vi "Measurement_WVFM.vi"(0 "dt":dbl, 2 "Input cluster":T1, 3 "Ioffset":dbl) -> (4 "Total power values":dbl[](array[numeric]), 5 "VL array":waveform(sgl)[](array[waveform]), 6 "VR array":waveform(sgl)[](array[waveform]), 7 "RMS values":dbl[](array[numeric]), 8 "Active Power":dbl[](array[numeric]))   [LabVIEW 2016]
uses:
  <vilib>/addons/Electrical Power/Basic/Measurement/RMS (N Channels).vi
  <vilib>/addons/Electrical Power/Basic/Measurement/Fundamental Vector (N Channels).vi
  <vilib>/addons/Electrical Power/Basic/NI_EP_Basic.lvlib
panel:
  out "RMS values I":dbl[](array[numeric])
  out "RMS values VR":dbl[](array[numeric])
  out "RMS values VL":dbl[](array[numeric])
  out "I array":waveform(sgl)[](array[waveform])
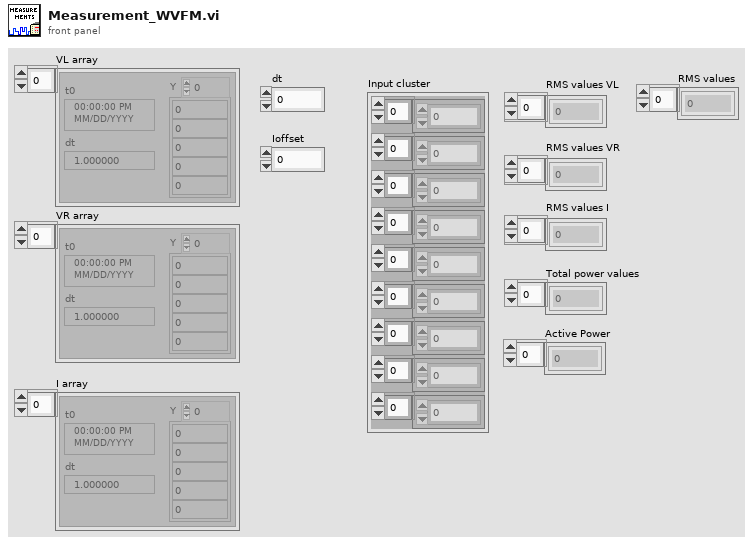
[diagram p1: front panel]
types:
  T1 = cluster{fxp<+/-,26,5>[], fxp<+/-,26,5>[], fxp<+/-,26,5>[], fxp<+/-,26,5>[], fxp<+/-,26,5>[], fxp<+/-,26,5>[], fxp<+/-,26,5>[], fxp<+/-,26,5>[], fxp<+/-,26,5>[]}
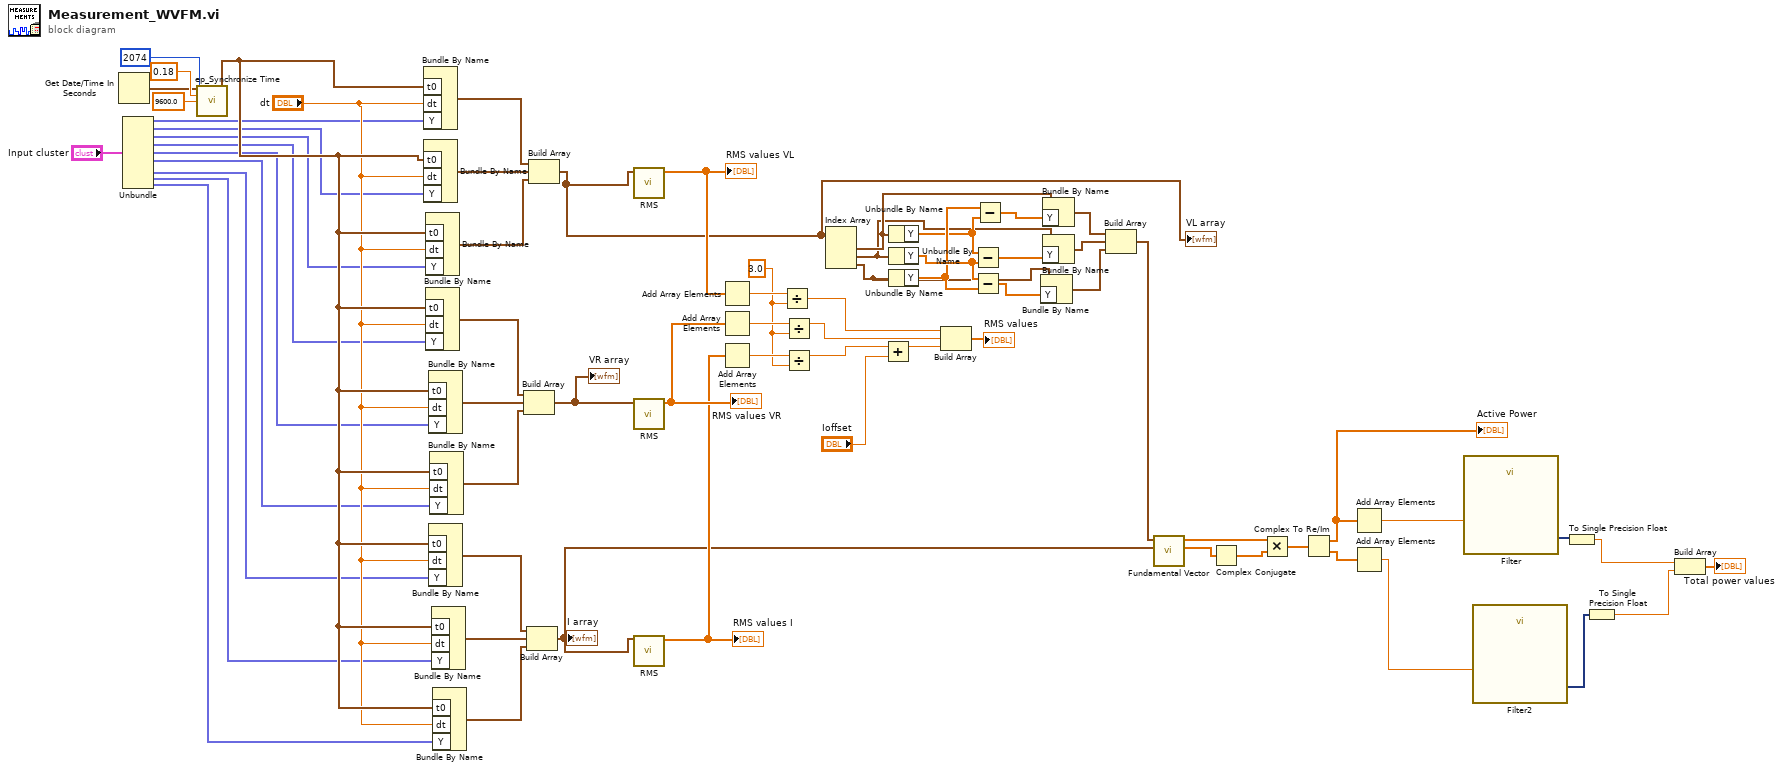
[diagram p0: block diagram]
diagram:
  w6 = 3.0 ("x")
  n1 = Get Date/Time In Seconds() -> (seconds since 1Jan1904=w58:timestamp)
  n2 = Unbundle("Input cluster") -> (w52:fxp<+/-,26,5>[], w51:fxp<+/-,26,5>[], w50:fxp<+/-,26,5>[], w49:fxp<+/-,26,5>[], w48:fxp<+/-,26,5>[], w47:fxp<+/-,26,5>[], w46:fxp<+/-,26,5>[], w45:fxp<+/-,26,5>[], w44:fxp<+/-,26,5>[])
  n3 = call <vilib>:"ep_Synchronize Time.vi"("RT controler time in"=w58, "maximum time difference (sec)"=0.18, "sampling rate (Hz)"=9600.0, "basic calc. interval (samples)"=2074) -> ("RT controler time out"=w55:timestamp)  [unwired: 11 in]
  n4 = Bundle By Name("t0"=w55, "dt"="dt", "Y"=w52) -> (w64:waveform(dbl))  [unwired: 1 in]
  n5 = Bundle By Name("t0"=w55, "dt"="dt", "Y"=w51) -> (w63:waveform(dbl))  [unwired: 1 in]
  n6 = Bundle By Name("t0"=w55, "dt"="dt", "Y"=w50) -> (w62:waveform(dbl))  [unwired: 1 in]
  n7 = Bundle By Name("t0"=w55, "dt"="dt", "Y"=w49) -> (w61:waveform(sgl))  [unwired: 1 in]
  n8 = Bundle By Name("t0"=w55, "dt"="dt", "Y"=w48) -> (w60:waveform(sgl))  [unwired: 1 in]
  n9 = Bundle By Name("t0"=w55, "dt"="dt", "Y"=w46) -> (w27:waveform(sgl))  [unwired: 1 in]
  n10 = Bundle By Name("t0"=w55, "dt"="dt", "Y"=w47) -> (w59:waveform(sgl))  [unwired: 1 in]
  n11 = Bundle By Name("t0"=w55, "dt"="dt", "Y"=w45) -> (w56:waveform(sgl))  [unwired: 1 in]
  n12 = Bundle By Name("t0"=w55, "dt"="dt", "Y"=w44) -> (w57:waveform(sgl))  [unwired: 1 in]
  n13 = Build Array(w61, w60, w59) -> (w43:waveform(sgl)[])
  "VR array" <- w43
  n14 = Build Array(w27, w56, w57) -> (w24:waveform(sgl)[])
  "I array" <- w24
  n15 = Build Array(w64, w63, w62) -> (w3:waveform(dbl)[])
  "VL array" <- w3
  n16 = call-poly <vilib>:"RMS.vi"("waveforms"=w3) -> ("RMS values"=w42:dbl[])  [unwired: 9 in, 1 out]
  "RMS values VL" <- w42
  n17 = call-poly <vilib>:"RMS.vi"("waveforms"=w43) -> ("RMS values"=w41:dbl[])  [unwired: 9 in, 1 out]
  "RMS values VR" <- w41
  n18 = call-poly <vilib>:"RMS.vi"("waveforms"=w24) -> ("RMS values"=w40:dbl[])  [unwired: 9 in, 1 out]
  "RMS values I" <- w40
  n19 = Add Array Elements(numeric array=w42) -> (sum=w12:dbl)
  n20 = Add Array Elements(numeric array=w41) -> (sum=w11:dbl)
  n21 = Add Array Elements(numeric array=w40) -> (sum=w10:dbl)
  n22 = Divide(x=w12, y=w6) -> (x/y=w9:dbl)
  n23 = Divide(x=w11, y=w6) -> (x/y=w8:dbl)
  n24 = Divide(x=w10, y=w6) -> (x/y=w7:dbl)
  n25 = Index Array(array=w3) -> (element #1=w35:waveform(dbl), element #2=w34:waveform(dbl), element #3=w32:waveform(dbl))  [unwired: 3 in]
  n26 = Add(x=w7, y="Ioffset") -> (x+y=w2:dbl)
  n27 = Unbundle By Name(w35) -> ("Y"=w37:dbl[])
  n28 = Unbundle By Name(w34) -> ("Y"=w39:dbl[])
  n29 = Unbundle By Name(w32) -> ("Y"=w38:dbl[])
  n30 = Build Array(w9, w8, w2) -> (→"RMS values":dbl[])
  n31 = Subtract(x=w37, y=w39) -> (x-y=w33:dbl[])
  n32 = Subtract(x=w39, y=w38) -> (x-y=w31:dbl[])
  n33 = Subtract(x=w38, y=w37) -> (x-y=w36:dbl[])
  n34 = Bundle By Name(cluster=w32, "Y"=w31) -> (w29:waveform(dbl))
  n35 = Bundle By Name(cluster=w35, "Y"=w36) -> (w28:waveform(dbl))
  n36 = Bundle By Name(cluster=w34, "Y"=w33) -> (w30:waveform(dbl))
  n37 = Build Array(w28, w30, w29) -> (w13:waveform(dbl)[])
  n38 = call-poly <vilib>:"Fundamental Vector.vi"("current waveforms"=w24, "voltage waveforms"=w13) -> ("current fundamental vectors"=w22:cdb[], "voltage fundamental vectors"=w23:cdb[])  [unwired: 6 in, 2 out]
  n39 = Complex Conjugate(1:w22) -> (0:w25:cdb[])
  n40 = Multiply(x=w23, y=w25) -> (x*y=w26:cdb[])
  n41 = Complex To Re/Im(x + iy=w26) -> (x=w21:dbl[], y=w20:dbl[])
  "Active Power" <- w21
  n42 = Add Array Elements(numeric array=w21) -> (sum=w16:dbl)
  n43 = Add Array Elements(numeric array=w20) -> (sum=w4:dbl)
  n44 = call "Filter"("Signal"=w16) -> ("Filtered Signal"=w18:dynamicdata)  [unwired: 9 in, 1 out]
  n45 = call "Filter2"("Signal"=w4) -> ("Filtered Signal"=w17:dynamicdata)  [unwired: 9 in, 1 out]
  n46 = To Single Precision Float(number=w18) -> (single precision float=w15:sgl)
  n47 = To Single Precision Float(number=w17) -> (single precision float=w14:sgl)
  n48 = Build Array(w15, w14) -> (→"Total power values":sgl[])
